vi "set address.source.vi"(6 "timeout (25000ms)":i32=25000, 8 "error in (no error)":errorcluster, 10 "address":i32=240 format="%02x", 11 "daemon reference in":refnum<k5>) -> (0 "error out":errorcluster, 2 "response":string, 3 "daemon reference out":refnum<k5>, 4 "parameter(s) out":string, 5 "command out":string="set_source_address")   [LabVIEW 2017]
doc: "<b>Command: </b>\"set_source_address\"\n\n<b>Description: </b> This command instructs the Daemon to change the DIPC source address.\n\n<b>Parameters: </b>\n\n 1. Source Address\n____________________________________________\nDIPC 692 Daemon API 10.0.0.1\nSam Tee - Dyson Technology Ltd\nCopyright (c) 2024, Dyson Technology Ltd"
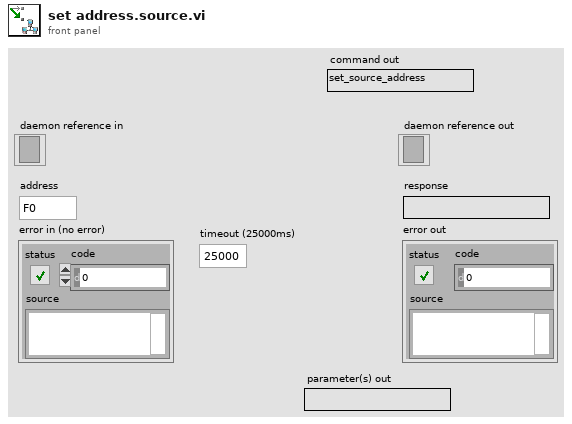
[diagram p1: front panel]
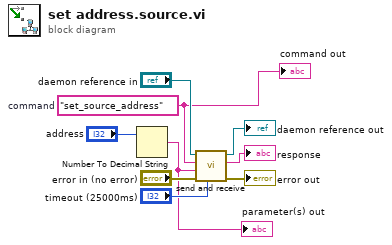
[diagram p0: block diagram]
diagram:
  w7 = "set_source_address"  # command
  n1 = Number To Decimal String(number="address") -> (decimal integer string=w1:string)  [unwired: 1 in]
  "parameter(s) out" <- w1
  n2 = call "send and receive.vi"("timeout (25000ms)"="timeout (25000ms)", "error in (no error)"="error in (no error)", "data"=w1, "command"=w7, "daemon reference in"="daemon reference in") -> ("error out"=→"error out":errorcluster, "response"=→"response":string, "daemon reference out"=→"daemon reference out":refnum<k5>)  [unwired: 4 in]
  "command out" <- w7
